vi "ArduinoStepMotor.vi"() -> ()   [LabVIEW 2024]
uses:
  <vilib>/MakerHub/LINX/Public/Peripherals/Digital/Digital Write 1 Chan.vi
  <vilib>/MakerHub/LINX/Public/Peripherals/PWM/PWM Set Duty Cycle 1 Chan.vi
  <vilib>/MakerHub/LINX/Public/Peripherals/Digital/Digital Write N Chans.vi
  <vilib>/MakerHub/LINX/Private/Local IO/LinxDigitalWrite.vi
  <vilib>/MakerHub/LINX/Public/Utilities/Check Channel.vi
  <vilib>/MakerHub/LINX/Public/Utilities/Open Serial.vi
  <vilib>/MakerHub/LINX/Private/Utilties/Generate Error.vi
  <vilib>/MakerHub/LINX/Public/Peripherals/PWM/PWM Set Duty Cycle N Chans.vi
  <vilib>/MakerHub/LINX/LMH-LINX.lvlib
panel:
  in  "Motor Speed":dbl(knob) scale=0.0..255.0
  in  "Serial Port":refnum<visa-resource-name>="N/A"
  in  "Motor Direction":bool
  in  "PWM Channel":u8
  in  "Motor Direction Pin 2":u8
  in  "Motor Direction Pin 1":u8
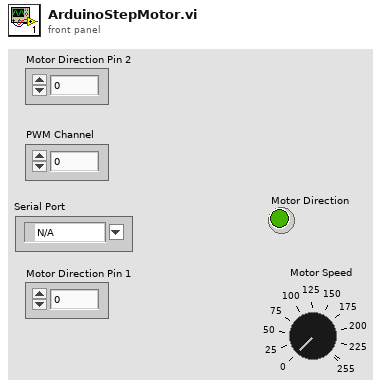
[diagram p1: front panel]
types:
  T1 = typedef "LMH-LINX.lvlib/LINX Ref.ctl" = cluster{"IO":T2, "Interface":T3, "LINX Device Config":T4}
  T2 = typedef "LMH-LINX.lvlib/Platform.ctl" = enum16{"Remote", "Local"}
  T3 = typedef "LMH-LINX.lvlib/Interface.ctl" = enum16{"Serial", "TCP"}
  T4 = typedef "LMH-LINX.lvlib/Device.lvlib/LINX Device Config.ctl" = cluster{"Interface":T3, "COM Port":refnum<visa-resource-name>, "TCP Configuration":T5, "Device Family":u8, "Device ID":u8, "Device Name":string, "TCP Ref":refnum<k5>, "Channels":T6}
  T5 = typedef "LMH-LINX.lvlib/Device.lvlib/TCP Config.ctl" = cluster{"IP Address":string, "Port":u16}
  T6 = typedef "LMH-LINX.lvlib/Channels.ctl" = cluster{"DI":u8[], "DO":u8[], "AI":u8[], "AO":u8[], "PWM":u8[], "QE":u8[], "UART":u8[], "I2C 2":u8[], "SPI":u8[], "CAN":u8[], "Servo":u8[], "AI Ref (V)":dbl, "AI Resolution (Bits)":u8, "AO Ref (V)":dbl, "AO Resolution (Bits)":u8}
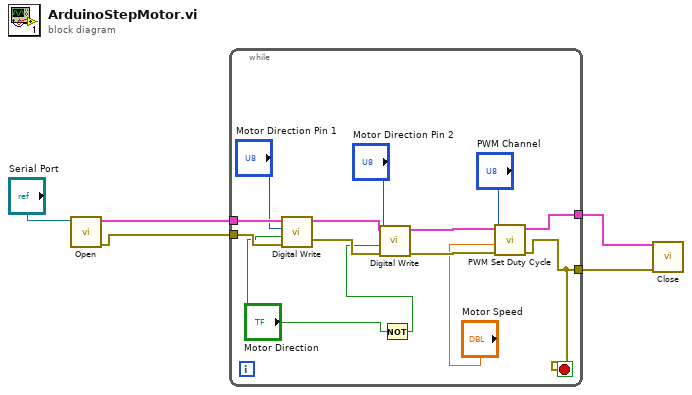
[diagram p0: block diagram]
diagram:
  n1 = call-poly <vilib>:"Open.vi"("Serial Port"="Serial Port") -> ("Error Out"=w3:errorcluster, "LINX Resource"=w5:T1)  [unwired: 8 in, 1 out]
  n2 = while {
    tunnel: w5 -> [w19]
    tunnel: [w17] -> w4
    tunnel: w3 -> [w16]
    tunnel: [w9] -> w2
    stop <- w9 stop-if-true
    n3 = call-poly <vilib>:"Digital Write.vi"("Error In"=w16, "Output Value"="Motor Direction", "DO Channel"="Motor Direction Pin 1", "LINX Resource"=w19) -> ("Error Out"=w15:errorcluster, "LINX Resource"=w13:T1)  [unwired: 6 in]
    n4 = Not(x="Motor Direction") -> (.not. x?=w7:bool)
    n5 = call-poly <vilib>:"Digital Write.vi"("Error In"=w15, "Output Value"=w7, "DO Channel"="Motor Direction Pin 2", "LINX Resource"=w13) -> ("Error Out"=w14:errorcluster, "LINX Resource"=w18:T1)  [unwired: 6 in]
    n6 = call-poly <vilib>:"PWM Set Duty Cycle.vi"("Error In"=w14, "Duty Cycle (0-1)"="Motor Speed", "PWM Channel"="PWM Channel", "LINX Resource"=w18) -> ("Error Out"=w9:errorcluster, "LINX Resource"=w17:T1)  [unwired: 6 in]
  }
  n7 = call <vilib>:"Close.vi"("Error In"=w2, "LINX Resource"=w4) -> ()  [unwired: 9 in, 1 out]
